vi "FlipstogramDual.vi"(4 "intervals":i32=22, 6 "Array2":dbl[](array[numeric]), 8 "Array1":dbl[](array[numeric])) -> (0 "Flipst2norm":cluster{"PDF(x)":i32[], "X Values":dbl[]}, 1 "Flipst2":T1, 2 "Flipst1norm":cluster{"PDF(x)":i32[], "X Values":dbl[]}, 3 "Flipst1":T1)   [LabVIEW 2016]
doc: "Produces 2 histograms, sharing common bins"
uses:
  <vilib>/Analysis/NI_AALPro.lvlib
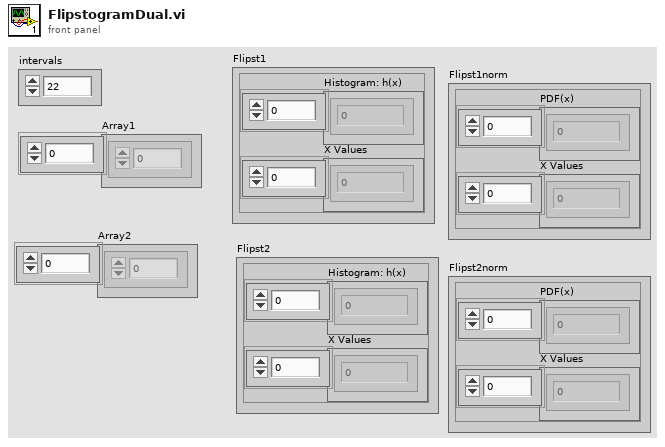
[diagram p1: front panel]
types:
  T1 = cluster{"Histogram: h(x)":i32[], "X Values":dbl[]}
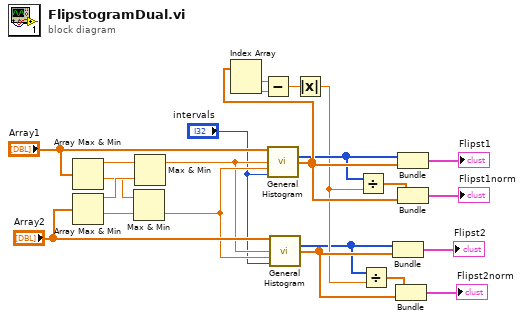
[diagram p0: block diagram]
diagram:
  n1 = Array Max & Min(array="Array1") -> (max value=w23:dbl, min value=w21:dbl)  [unwired: 2 out]
  n2 = Array Max & Min(array="Array2") -> (max value=w22:dbl, min value=w20:dbl)  [unwired: 2 out]
  n3 = Max & Min(x=w21, y=w20) -> (min(x,y)=w17:dbl)  [unwired: 1 out]
  n4 = Max & Min(x=w23, y=w22) -> (max(x,y)=w16:dbl)  [unwired: 1 out]
  n5 = call <vilib>:"General Histogram.vi"("X"="Array1", "max"=w16, "min"=w17, "# bins"="intervals") -> ("Histogram"=w7:i32[], "Axis"=w8:dbl[])  [unwired: 7 in, 3 out]
  n6 = Index Array(array=w8) -> (element #1=w12:dbl, element #2=w11:dbl)  [unwired: 2 in]
  n7 = Subtract(x=w12, y=w11) -> (x-y=w10:dbl)
  n8 = call <vilib>:"General Histogram.vi"("X"="Array2", "max"=w16, "min"=w17, "# bins"="intervals") -> ("Histogram"=w2:i32[], "Axis"=w4:dbl[])  [unwired: 7 in, 3 out]
  n9 = Absolute Value(x=w10) -> (abs(x)=w3:dbl)
  n10 = Divide(x=w7, y=w3) -> (x/y=w6:dbl[])
  n11 = Divide(x=w2, y=w3) -> (x/y=w1:dbl[])
  n12 = Bundle("Histogram"=w2, "Axis"=w4) -> (→"Flipst2":cluster{"Histogram":i32[], "Axis":dbl[]})  [unwired: 1 in]
  n13 = Bundle(w1, "Axis"=w4) -> (→"Flipst2norm":cluster{dbl[], "Axis":dbl[]})  [unwired: 1 in]
  n14 = Bundle("Histogram"=w7, "Axis"=w8) -> (→"Flipst1":cluster{"Histogram":i32[], "Axis":dbl[]})  [unwired: 1 in]
  n15 = Bundle(w6, "Axis"=w8) -> (→"Flipst1norm":cluster{dbl[], "Axis":dbl[]})  [unwired: 1 in]
